vi "write text file.vi"(8 "error in":errorcluster, 10 "text":string, 11 "file path in":path) -> (0 "error out":errorcluster, 3 "path out":path)   [LabVIEW 2023, in "Reusable Library.lvlib"]
uses:
  Reusable Library.lvlib
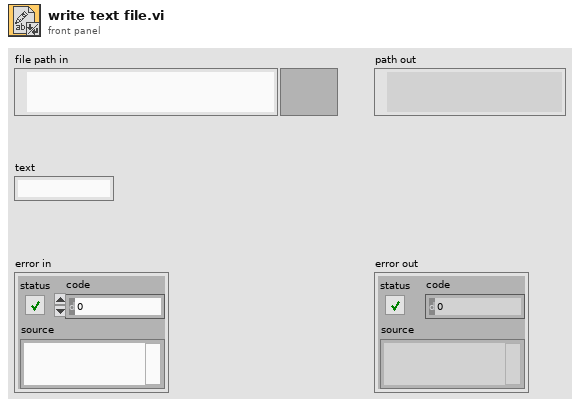
[diagram p1: front panel]
types:
  T1 = enum16{"open", "replace", "create", "open or create", "replace or create", "replace or create with confirmation"}
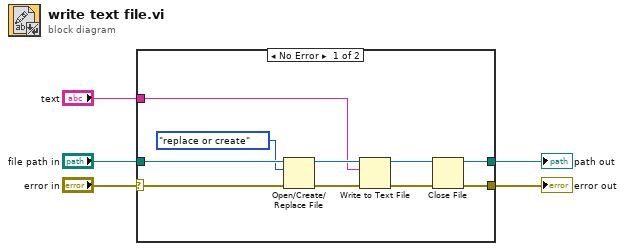
[diagram p0: block diagram]
diagram:
  n1 = case shown="No Error" "error in" {
    selector: "error in" -> [w7 w16]
    tunnel: "text" -> [w11 _]
    tunnel: "file path in" -> [w10 w17]
    tunnel: [w9 w17] -> w3
    tunnel: [w8 w16] -> w2
    frame No Error {
      n2 = Open/Create/Replace File(file path (use dialog)=w10, error in=w7, operation (0:open)=T1."replace or create") -> (refnum out=w15:refnum<file>, error out=w13:errorcluster)  [unwired: 3 in, 1 out]
      n3 = Write to Text File(file (use dialog)=w15, text=w11, error in=w13) -> (refnum out=w14:refnum<file>, error out=w12:errorcluster)  [unwired: 1 in, 1 out]
      n4 = Close File(refnum=w14, error in=w12) -> (path=w9:path, error out=w8:errorcluster)
    }
    frame Error {
    }
  }
  "path out" <- w3
  "error out" <- w2
